vi "UploadYBRigolRAP.vi"(9 "OP Time":dbl, 10 "1762 Pulse Time":dbl, 11 "1762 Frequency":dbl) -> ()   [LabVIEW 2009]
panel:
  out "error out":errorcluster
  out "Command String":string
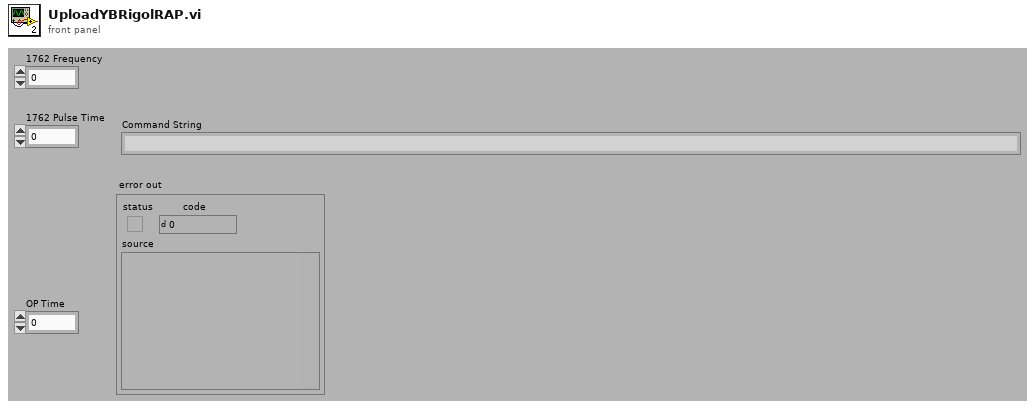
[diagram p1: front panel]
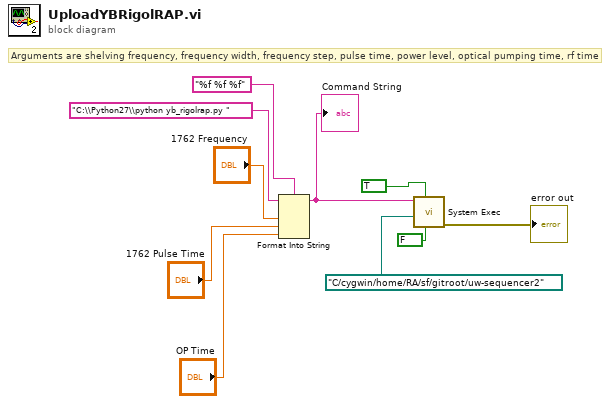
[diagram p0: block diagram]
diagram:
  # "Arguments are shelving frequency, frequency width, frequency step, pulse time, power level, optical pumping time, rf time"
  n1 = Format Into String(format string="%f %f %f" ("initial string"), initial string="C:\\Python27\\python yb_rigolrap.py " ("input 1"), "1762 Frequency", "1762 Pulse Time", "OP Time") -> (resulting string=w9:string)  [unwired: 1 in, 1 out]
  "Command String" <- w9
  n2 = call <vilib>:"System Exec.vi"("run minimized? (F)"=FALSE, "wait until completion? (T)"=TRUE, "working directory"=path "C:/cygwin/home/RA/sf/gitroot/uw-sequencer2", "command line"=w9) -> ("error out"=→"error out":errorcluster)  [unwired: 4 in, 3 out]
